vi "BKPrecision_PS_Control.vi"(6 "Current Limit (0)":dbl=3.0 min=0.0 max=6.0 format="%#.2g", 7 "Output on/off":bool, 8 "error in (no error)":errorcluster, 9 "Output Voltage (0)":dbl min=0.0 max=31.0 format="%#.2f", 10 "Maximum Output Voltage (31)":dbl=31.0 min=0.0 max=31.0 format="%#.2f", 11 "VISA resource name":refnum<visa-resource-name>) -> (0 "error out":errorcluster, 3 "VISA resource name out":refnum<visa-resource-name>)   [LabVIEW 2015]
uses:
  <instrlib>/BK Precision 178XB Series/BK Precision 178XB Series.lvlib
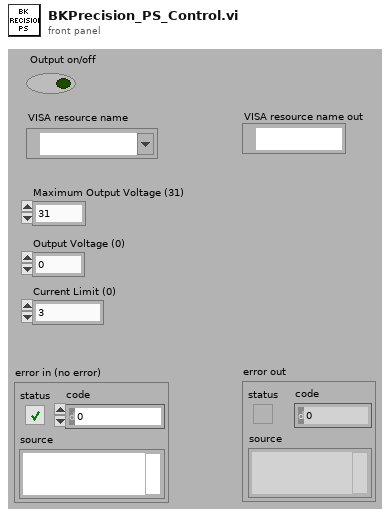
[diagram p1: front panel]
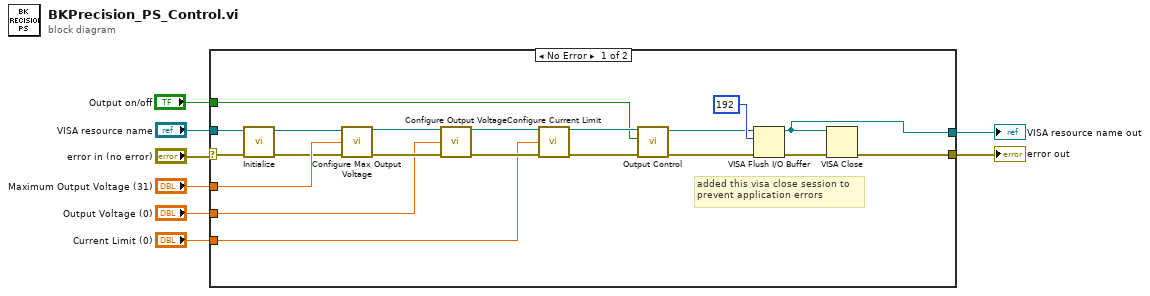
[diagram p0: block diagram]
diagram:
  n1 = case shown="No Error" "error in (no error)" {
    selector: "error in (no error)" -> [w10 w30]
    tunnel: "Maximum Output Voltage (31)" -> [w22 _]
    tunnel: "Output Voltage (0)" -> [w21 _]
    tunnel: "Current Limit (0)" -> [w20 _]
    tunnel: [w15 w30] -> w5
    tunnel: "VISA resource name" -> [w12 w29]
    tunnel: [w14 w29] -> w3
    tunnel: "Output on/off" -> [w13 _]
    frame No Error {
      # "added this visa close session to \nprevent application errors"
      n2 = call <instrlib>:"Initialize.vi"("error in (no error)"=w10, "VISA resource name"=w12) -> ("error out"=w9:errorcluster, "VISA resource name out"=w11:refnum<visa-resource-name>)  [unwired: 8 in]
      n3 = call <instrlib>:"Configure Max Output Voltage.vi"("VISA resource name"=w11, "Maximum Output Voltage (18)"=w22, "error in (no error)"=w9) -> ("VISA resource name out"=w28:refnum<visa-resource-name>, "error out"=w25:errorcluster)  [unwired: 11 in]
      n4 = call <instrlib>:"Configure Output Voltage.vi"("VISA resource name"=w28, "Output Voltage (0)"=w21, "error in (no error)"=w25) -> ("VISA resource name out"=w27:refnum<visa-resource-name>, "error out"=w26:errorcluster)  [unwired: 11 in]
      n5 = call <instrlib>:"Configure Current Limit.vi"("VISA resource name"=w27, "Current Limit (0)"=w20, "error in (no error)"=w26) -> ("VISA resource name out"=w24:refnum<visa-resource-name>, "error out"=w23:errorcluster)  [unwired: 11 in]
      n6 = call <instrlib>:"Output Control.vi"("error in (no error)"=w23, "Enable Output Terminals (F: Off)"=w13, "VISA resource name"=w24) -> ("error out"=w16:errorcluster, "VISA resource name out"=w17:refnum<visa-resource-name>)  [unwired: 7 in]
      n7 = VISA Flush I/O Buffer(VISA resource name=w17, mask (16)=u16 192, error in (no error)=w16) -> (VISA resource name out=w14:refnum<visa-resource-name>, error out=w19:errorcluster)
      n8 = VISA Close(VISA resource name=w14, error in (no error)=w19) -> (error out=w15:errorcluster)
    }
    frame Error {
    }
  }
  "error out" <- w5
  "VISA resource name out" <- w3
